vi "Config-front panel.vi"(8 "error in (no error)":errorcluster, 11 "CAP-USB-1 in":refnum<class "CAP-USB-1.lvclass">) -> (0 "error out":errorcluster, 2 "output cluster":T1, 3 "CAP-USB-1 out":refnum<class "CAP-USB-1.lvclass">)   [LabVIEW 2014, in "CAP-USB-1.lvlib" / "CAP-USB-1.lvclass"]
doc: "VI encargado de ejecutar el proceso de configuracion de los parametros del equipo"
uses:
  CAP-USB-1.lvclass
  DriverMasterSync/build/DriverMasterSync.lvlibp/Modules/HAL/TypeDefs/HAL Config Data.ctl
  CAP-USB-1.lvclass/CAP-USB-1.ctl
  DriverMasterSync/build/DriverMasterSync.lvlibp/Modules/HAL/DriverMasterSync/DriverMasterSyncClass/DriverMasterSync.lvclass
  DriverMasterSync/build/DriverMasterSync.lvlibp
panel:
  in  "Proteccion":bool
  in  "Offset":bool
  in  "Ganancia":bool
  in  "Transductores":bool
  in  "Reduccion":sgl=1.0
  in  "Muestras Diag. Cycle":u32=10
  in  "Tolerancia Cycle":sgl=5.0 caption="Tolerancia % Cycle"
  in  "Seleccion de Puerto COM":refnum<visa-resource-name>="COM3"
  in  "Delay Auto-Refresh(uS)":i32=30000
  in  "N° Tramas - Sequence":u32=90
  in  "Tolerancia":sgl=10.0 caption="Tolerancia %"
  in  "Pulsos Encoder":u16=3600
  in  "Delay Sequence(uS)":i32
  in  "Cancel":bool
  in  "OK":bool
  # "Guardar?"
  # "Salir?"
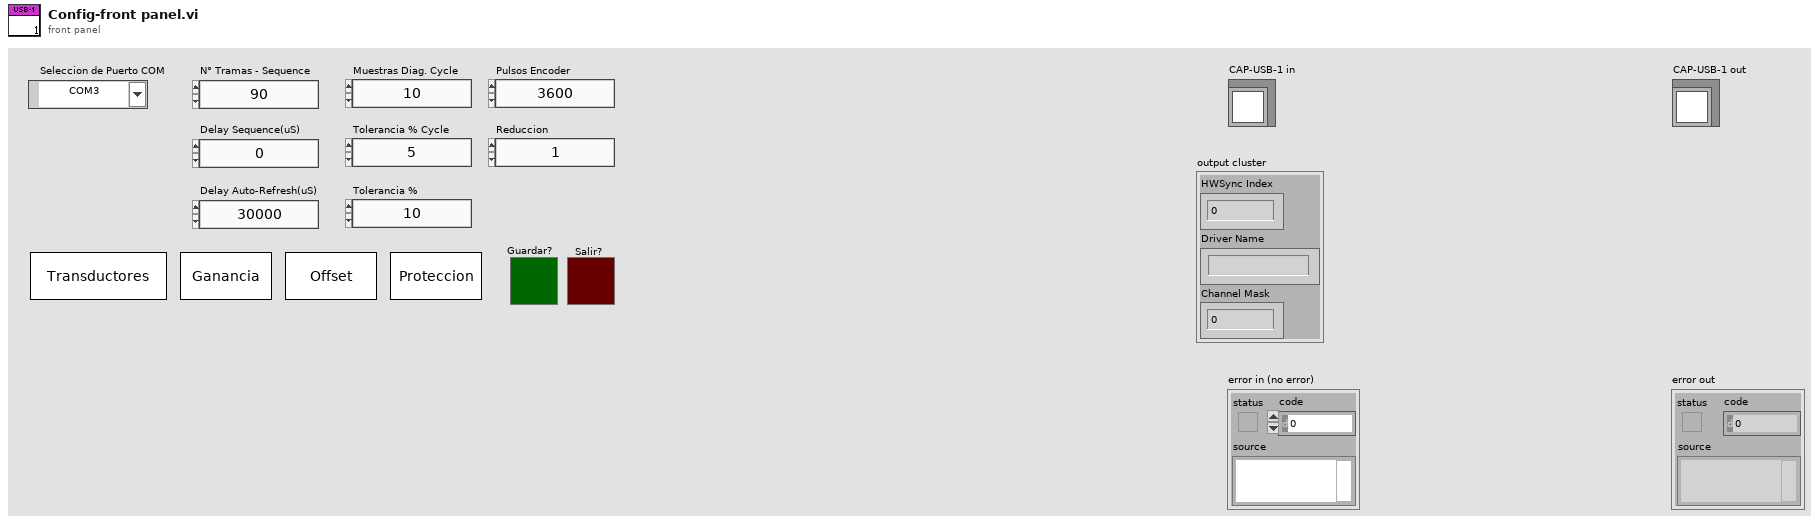
[diagram p1: front panel]
types:
  T1 = typedef "DriverMasterSync.lvlibp/HAL Config Data.ctl" = cluster{"HWSync Index":u32, "Driver Name":string, "Channel Mask":u64}
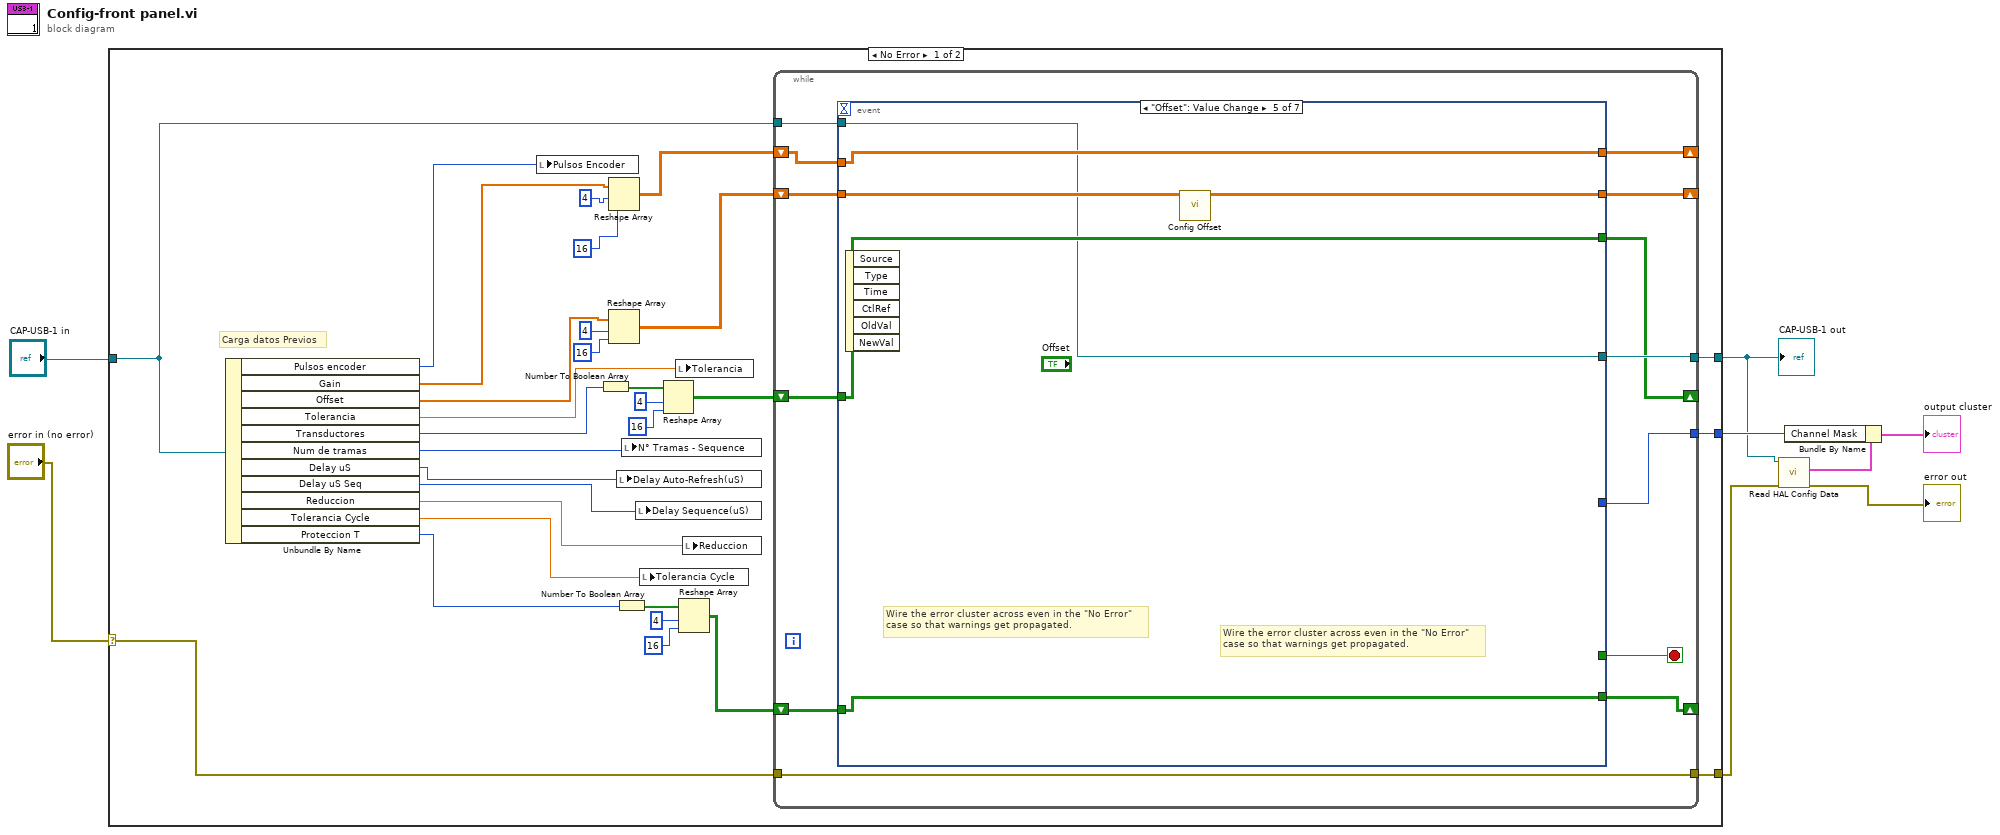
[diagram p0: block diagram]
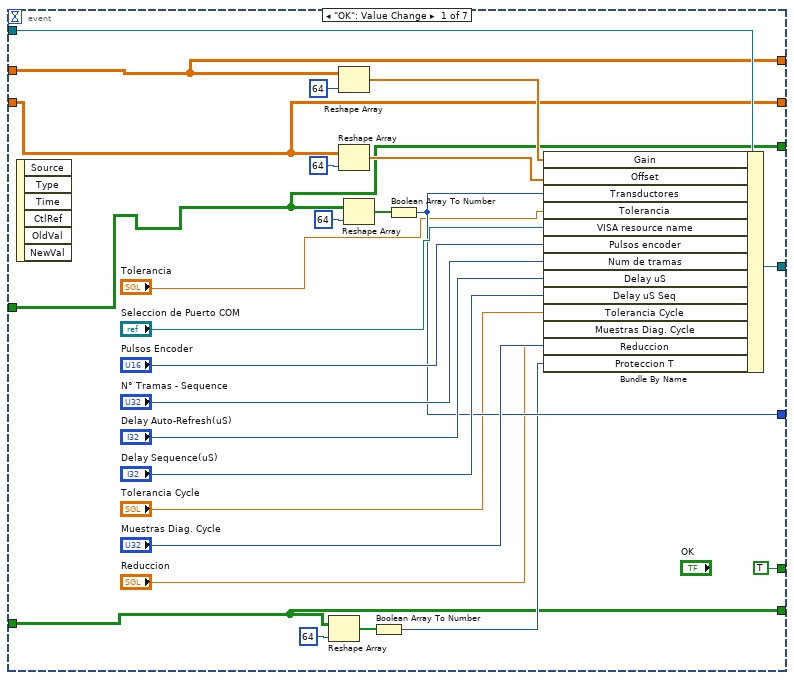
[diagram p2: hidden frame]
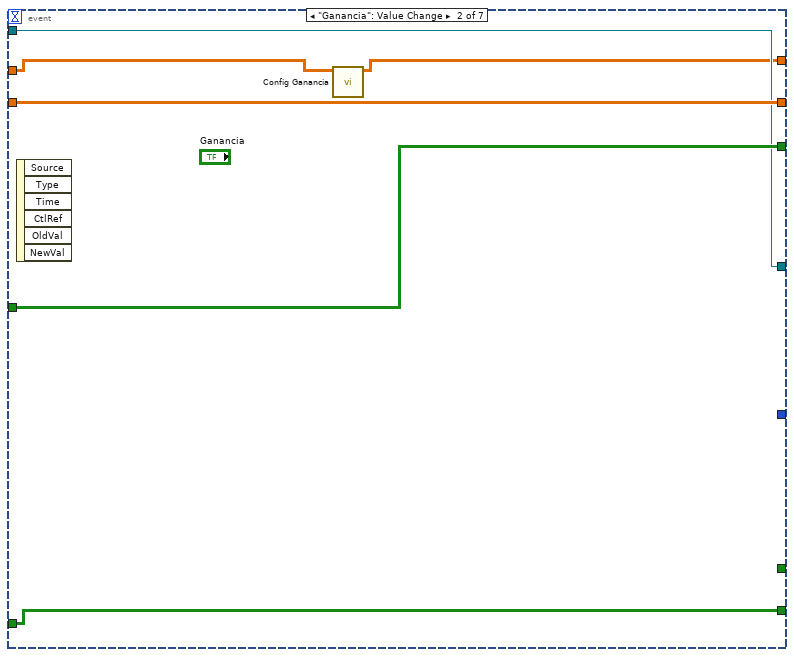
[diagram p3: hidden frame]
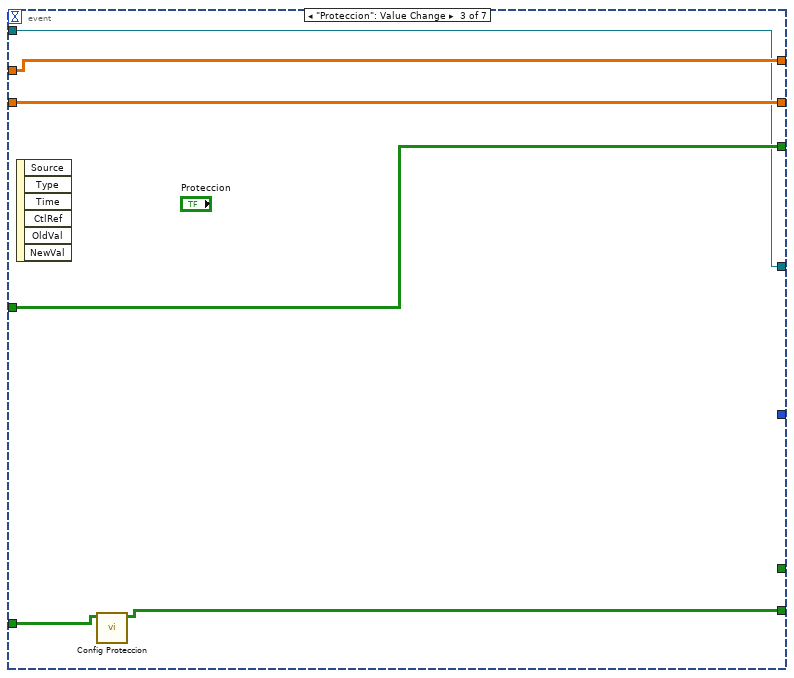
[diagram p4: hidden frame]
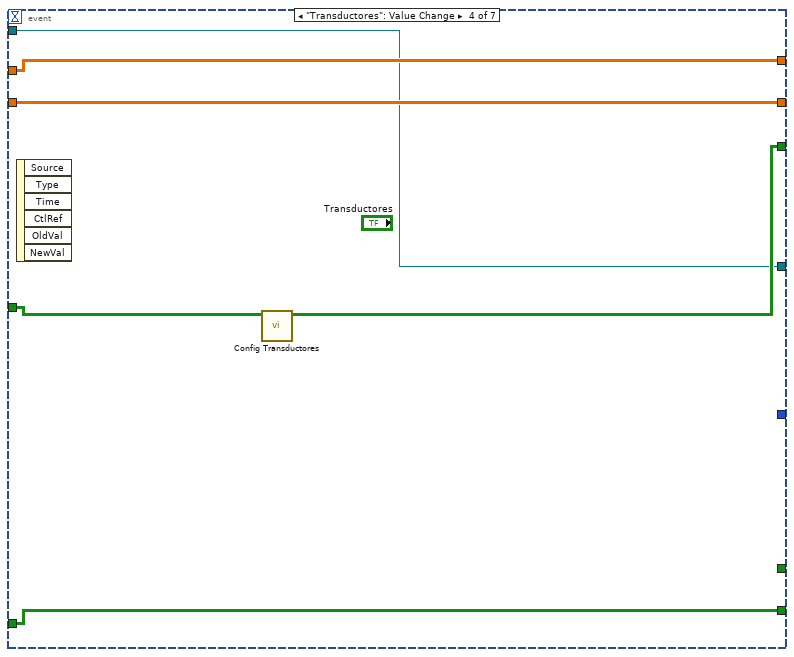
[diagram p5: hidden frame]
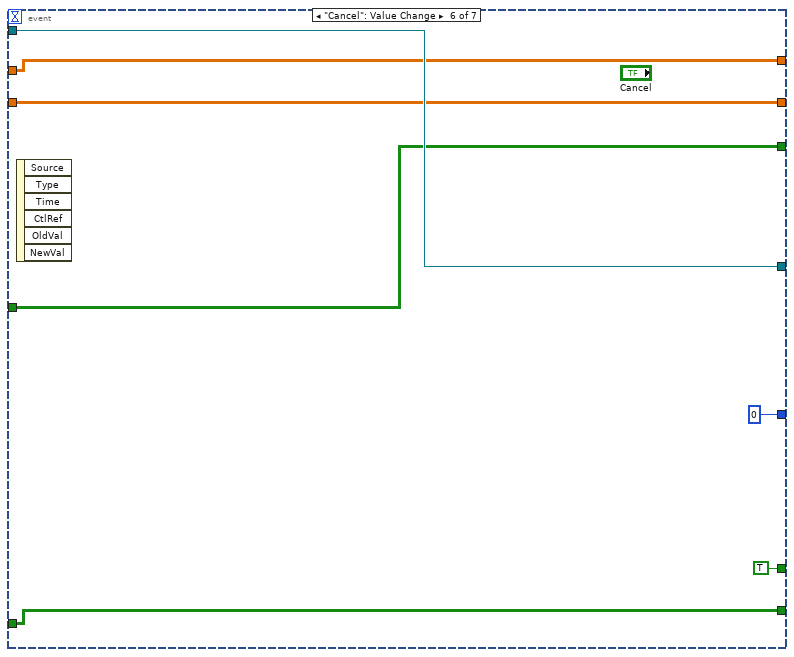
[diagram p6: hidden frame]
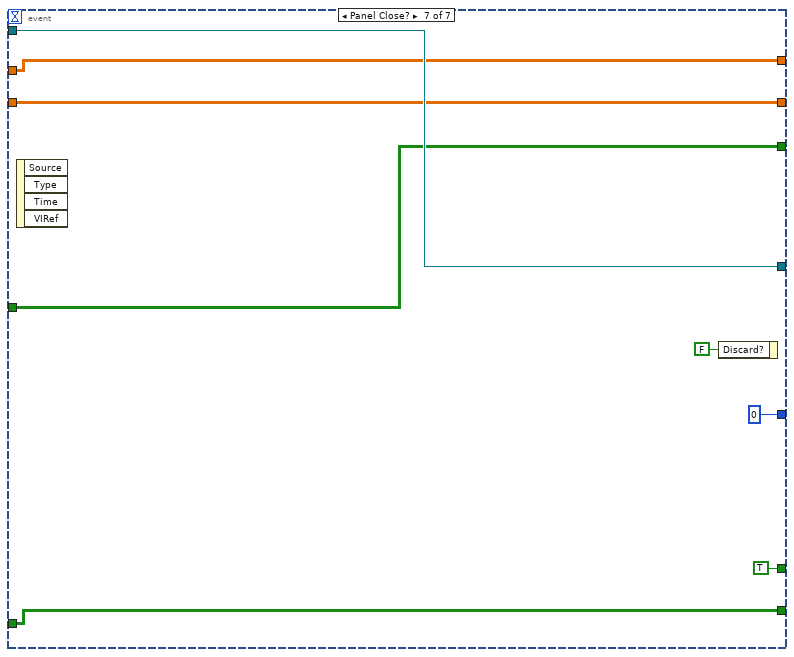
[diagram p7: hidden frame]
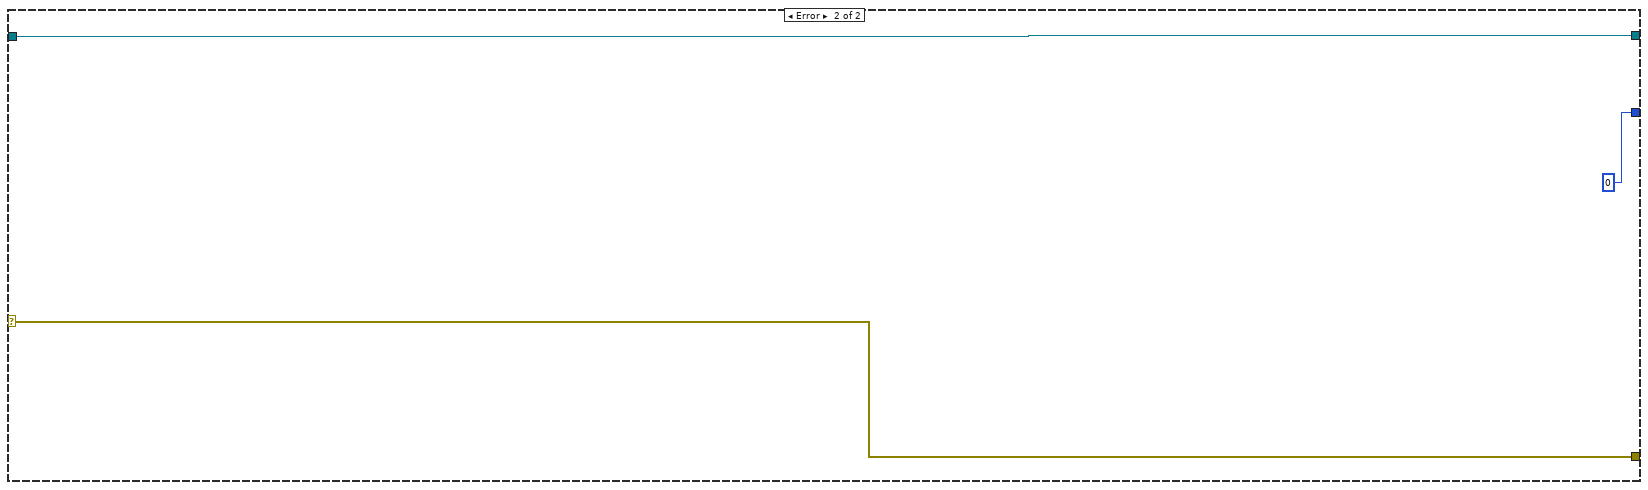
[diagram p8: hidden frame]
diagram:
  n1 = case shown="No Error" "error in (no error)" {
    selector: "error in (no error)" -> [w30 w119]
    tunnel: [w29 w119] -> w5
    tunnel: [w26 w118] -> w1
    tunnel: "CAP-USB-1 in" -> [w34 w118]
    tunnel: [w21 u64 0] -> w6
    frame No Error {
      # "Carga datos Previos"
      # "Wire the error cluster across even in the \"No Error\"\ncase so that warnings get propagated."
      # "Wire the error cluster across even in the \"No Error\"\ncase so that warnings get propagated."
      n2 = Unbundle By Name(w34) -> ("Pulsos encoder"=w11:u16, "Gain"=w36:sgl[], "Offset"=w35:sgl[], "Tolerancia"=w25:sgl, "Transductores"=w10:u64, "Num de tramas"=w24:u32, "Delay uS"=w23:i32, "Delay uS Seq"=w22:i32, "Reduccion"=w20:sgl, "Tolerancia Cycle"=w19:sgl, "Proteccion T"=w15:u64)
      n3 = local write "Pulsos Encoder"(w11) -> ()
      n4 = Number To Boolean Array(number=w10) -> (Boolean array=w33:bool[])
      n5 = Reshape Array(w36, 4 ("dimension size"), 16 ("dimension size")) -> (w13:sgl[][])
      n6 = Reshape Array(w35, 4 ("dimension size"), 16 ("dimension size")) -> (w12:sgl[][])
      n7 = local write "Delay Auto-Refresh(uS)"(w23) -> ()
      n8 = Number To Boolean Array(number=w15) -> (Boolean array=w18:bool[])
      n9 = local write "N° Tramas - Sequence"(w24) -> ()
      n10 = local write "Delay Sequence(uS)"(w22) -> ()
      n11 = local write "Tolerancia Cycle"(w19) -> ()
      n12 = Reshape Array(w33, 4 ("dimension size"), 16 ("dimension size")) -> (w9:bool[][])
      n13 = local write "Tolerancia"(w25) -> ()
      n14 = Reshape Array(w18, 4 ("dimension size"), 16 ("dimension size")) -> (w14:bool[][])
      n15 = local write "Reduccion"(w20) -> ()
      n16 = while {
        tunnel: w34 -> [w51]
        tunnel: [w50] -> w26
        tunnel: w30 -> [w48]
        tunnel: [w48] -> w29
        tunnel: [w47] -> w21
        shift-right: [w44] -> _
        shift-left: w13 -> [w43]
        shift-right: [w41] -> _
        shift-left: w12 -> [w46]
        shift-right: [w40] -> _
        shift-left: w9 -> [w42]
        shift-right: [w39] -> _
        shift-left: w14 -> [w45]
        stop <- w49 stop-if-true
        n17 = event shown="[4] \"Offset\": Value Change" {
          selector: _ -> [_ _ _ _ _ _ _]
          dyn-events: _ -> [_ _ _ _ _ _ _]
          timeout: _ -> [_ _ _ _ _ _ _]
          tunnel: [w77 w81 w84 w90 w96 w108 w116] -> w50
          tunnel: [TRUE ("OK") _ _ _ _ TRUE ("OK") TRUE ("OK")] -> w49
          tunnel: w51 -> [w72 w81 w84 w90 w96 w108 w116]
          tunnel: [w63 _ _ _ _ u64 0 u64 0] -> w47
          tunnel: w43 -> [w61 w80 w87 w93 w101 w105 w113]
          tunnel: w46 -> [w60 w83 w86 w92 w98 w106 w114]
          tunnel: w45 -> [w55 w78 w89 w91 w99 w104 w112]
          tunnel: [w61 w79 w87 w93 w101 w105 w113] -> w44
          tunnel: w42 -> [w56 w82 w85 w95 w100 w107 w115]
          tunnel: [w60 w83 w86 w92 w97 w106 w114] -> w41
          tunnel: [w56 w82 w85 w94 w100 w107 w115] -> w40
          tunnel: [w55 w78 w88 w91 w99 w104 w112] -> w39
          event "OK": Value Change {
            n18 = event-data() -> ()  [unwired: 1 in, 6 out]
            n19 = Reshape Array(w55, 64 ("dimension size")) -> (w58:bool[])
            n20 = Reshape Array(w61, 64 ("dimension size")) -> (w74:sgl[])
            n21 = Reshape Array(w60, 64 ("dimension size")) -> (w73:sgl[])
            n22 = Reshape Array(w56, 64 ("dimension size")) -> (w70:bool[])
            n23 = Boolean Array To Number(Boolean array=w58) -> (number=w57:u64)
            n24 = Boolean Array To Number(Boolean array=w70) -> (number=w63:u64)
            n25 = Bundle By Name(cluster=w72, "Gain"=w74, "Offset"=w73, "Transductores"=w63, "Tolerancia"="Tolerancia", "VISA resource name"="Seleccion de Puerto COM", "Pulsos encoder"="Pulsos Encoder", "Num de tramas"="N° Tramas - Sequence", "Delay uS"="Delay Auto-Refresh(uS)", "Delay uS Seq"="Delay Sequence(uS)", "Tolerancia Cycle"="Tolerancia Cycle", "Muestras Diag. Cycle"="Muestras Diag. Cycle", "Reduccion"="Reduccion", "Proteccion T"=w57) -> (w77:refnum<class "CAP-USB-1.lvclass">)
          }
          event "Ganancia": Value Change {
            n26 = event-data() -> ()  [unwired: 1 in, 6 out]
            n27 = call "Config Ganancia.vi"("Gain"=w80) -> ("Gain Out"=w79:sgl[][])  [unwired: 10 in]
          }
          event "Proteccion": Value Change {
            n28 = event-data() -> ()  [unwired: 1 in, 6 out]
            n29 = call "Config Proteccion.vi"("Transductores"=w89) -> ("Transductores Out"=w88:bool[][])  [unwired: 10 in]
          }
          event "Transductores": Value Change {
            n30 = event-data() -> ()  [unwired: 1 in, 6 out]
            n31 = call "Config Transductores.vi"("Transductores"=w95) -> ("Transductores Out"=w94:bool[][])  [unwired: 10 in]
          }
          event "Offset": Value Change {
            n32 = event-data() -> ()  [unwired: 1 in, 6 out]
            n33 = call "Config Offset.vi"("Offset"=w98) -> ("Offset Out"=w97:sgl[][])  [unwired: 10 in]
          }
          event "Cancel": Value Change {
            n34 = event-data() -> ()  [unwired: 1 in, 6 out]
          }
          event Panel Close? {
            n35 = event-data() -> ()  [unwired: 1 in, 4 out]
            n36 = event-data("Discard?"=FALSE) -> ()  [unwired: 1 in, 1 out]
          }
        }
      }
    }
    frame Error {
    }
  }
  "CAP-USB-1 out" <- w1
  n37 = call "Read HAL Config Data.vi"("error in (no error)"=w5, "DriverMasterSync in"=w1) -> ("error out"=→"error out":errorcluster, "HAL Config Data"=w8:T1)  [unwired: 7 in, 1 out]
  n38 = Bundle By Name(cluster=w8, "Channel Mask"=w6) -> (→"output cluster":T1)
